vi "Tree Tag Array to Full Names Array.vi"(11 "Selected Items Tags":string[](array[string])) -> (0 "Unnamed?":bool, 1 "Selected Item Indices":u32[](array[numeric]), 2 "size":i32, 3 "Tree Item Values (nested form)":cluster{"Array":string[]}[](array[cluster]), 5 "Display Names":string[](array[string]))   [LabVIEW 2023]
doc: "Convert the tree item tag values for each cluster item (dot-delimited) to the format required by the scripting node for bundle and unbundle (array or clluster of array of nested heirarchy)."
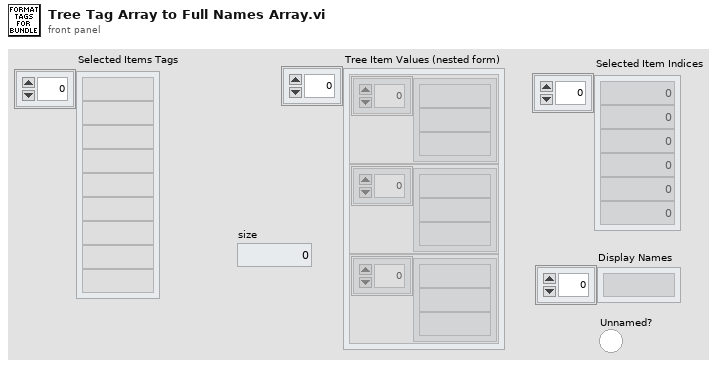
[diagram p1: front panel]
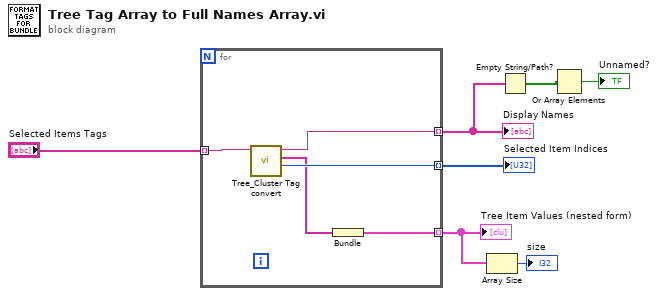
[diagram p0: block diagram]
diagram:
  n1 = for {
    tunnel: "Selected Items Tags" -> [w12] mode=indexing
    tunnel: [w8] -> w6 mode=indexing
    tunnel: [w10] -> w4 mode=indexing
    tunnel: [w11] -> w3 mode=indexing
    n2 = call "Tree_Cluster Tag convert.vi"("Tag"=w12) -> ("Index"=w10:u32, "Tree Nest"=w9:string[], "Display Name"=w11:string)  [unwired: 5 in, 3 out]
    n3 = Bundle("Tree Nest"=w9) -> (w8:cluster{"Tree Nest":string[]})  [unwired: 1 in]
  }
  "Tree Item Values (nested form)" <- w6
  "Selected Item Indices" <- w4
  "Display Names" <- w3
  n4 = Array Size(array=w6) -> (size(s)=→"size":i32)
  n5 = Empty String/Path?(string/path=w3) -> (empty?=w2:bool[])
  n6 = Or Array Elements(Boolean array=w2) -> (logical OR=→"Unnamed?":bool)
